vi "Log commands.vi"(7 "Log destination":T1, 8 "error in":errorcluster, 11 "text to log":string) -> (0 "error out":errorcluster)   [LabVIEW 2019]
doc: "Nicolas Weiss - EPFL - IPHYS 2019\n----\nThis VI logs text either to the User Interface or to file (or both)."
uses:
  Controls/Log destination selector.ctl
  _Global variables 1.vi
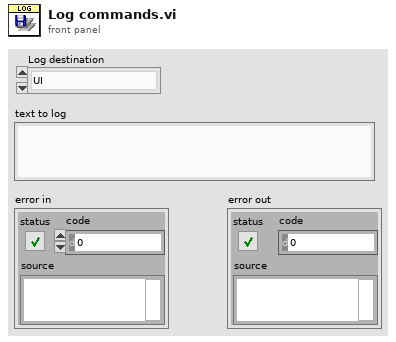
[diagram p1: front panel]
types:
  T1 = typedef "Log destination selector.ctl" = enum16{"UI", "File", "UI+file"}
  T2 = enum16{"open", "replace", "create", "open or create", "replace or create", "replace or create with confirmation"}
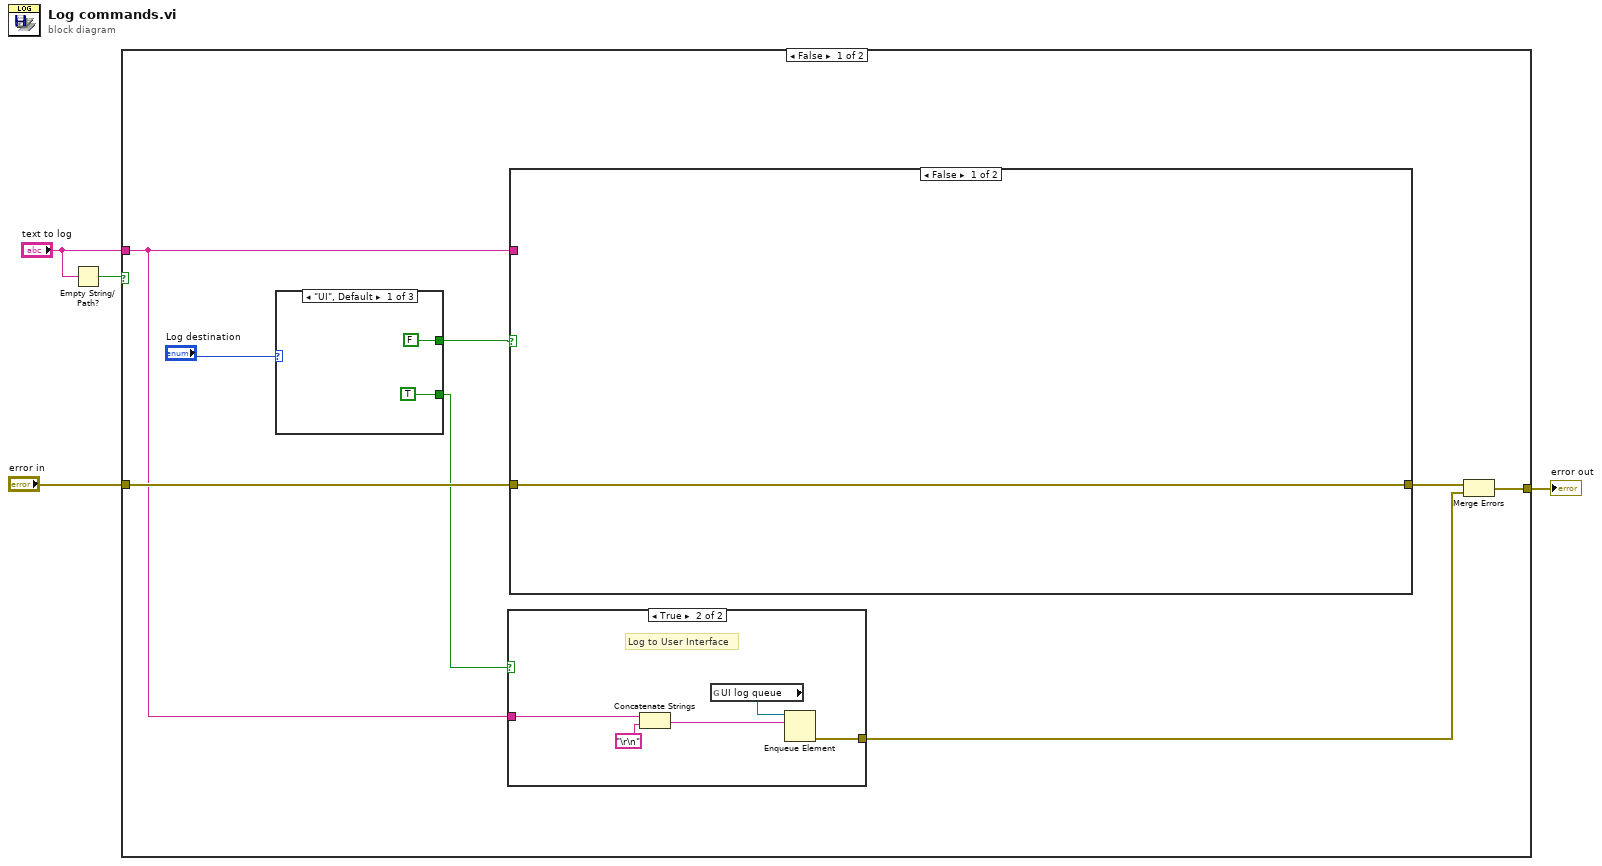
[diagram p0: block diagram]
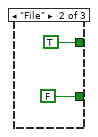
[diagram p3: hidden frame]
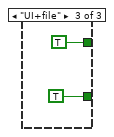
[diagram p4: hidden frame]
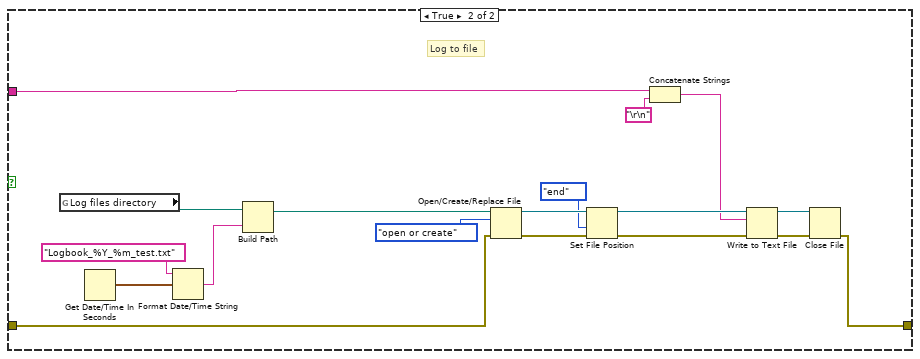
[diagram p5: hidden frame]
diagram:
  n1 = Empty String/Path?(string/path="text to log") -> (empty?=w1:bool)
  n2 = case shown="False" w1 {
    tunnel: "error in" -> [w12 w43]
    tunnel: [w5 w43] -> w3
    tunnel: "text to log" -> [w8 _]
    frame False {
      n3 = case shown="\"UI\", Default" "Log destination" {
        tunnel: [FALSE TRUE TRUE] -> w10
        tunnel: [TRUE FALSE TRUE] -> w9
        frame "UI", Default {
        }
        frame "File" {
        }
        frame "UI+file" {
        }
      }
      n4 = case shown="True" w9 {
        tunnel: w8 -> [_ w16]
        tunnel: [_ w13] -> w6
        frame False {
        }
        frame True {
          # "Log to User Interface"
          n5 = Concatenate Strings(w16, "\r\n") -> (w15:string)
          n6 = global read "_Global variables 1.vi" "UI log queue"() -> (w14:refnum<queue>)
          n7 = Enqueue Element(queue=w14, element=w15) -> (error out=w13:errorcluster)  [unwired: 2 in, 2 out]
        }
      }
      n8 = case shown="False" w10 {
        tunnel: w12 -> [w24 w37]
        tunnel: [w24 w36] -> w7
        tunnel: w8 -> [_ w35]
        frame False {
        }
        frame True {
          # "Log to file"
          n9 = global read "_Global variables 1.vi" "Log files directory"() -> (w42:path)
          n10 = Get Date/Time In Seconds() -> (seconds since 1Jan1904=w40:timestamp)
          n11 = Format Date/Time String(time format string (%c)="Logbook_%Y_%m_test.txt", seconds (now)=w40) -> (date/time string=w39:string)  [unwired: 1 in]
          n12 = Build Path(base path=w42, name or relative path=w39) -> (appended path=w38:path)
          n13 = Open/Create/Replace File(file path (use dialog)=w38, error in=w37, operation (0:open)=T2."open or create") -> (refnum out=w31:refnum<file>, error out=w29:errorcluster)  [unwired: 3 in, 1 out]
          n14 = Set File Position(refnum=w31, from (0:start)=enum16{"start", "end", "current"}."end", error in=w29) -> (refnum out=w30:refnum<file>, error out=w28:errorcluster)  [unwired: 1 in]
          n15 = Concatenate Strings(w35, "\r\n") -> (w25:string)
          n16 = Write to Text File(file (use dialog)=w30, text=w25, error in=w28) -> (refnum out=w33:refnum<file>, error out=w32:errorcluster)  [unwired: 1 in, 1 out]
          n17 = Close File(refnum=w33, error in=w32) -> (error out=w36:errorcluster)  [unwired: 1 out]
        }
      }
      n18 = Merge Errors(w7, w6) -> (w5:errorcluster)
    }
    frame True {
    }
  }
  "error out" <- w3
